vi "fft_test.vi"() -> ()   [LabVIEW 2012]
uses:
  <vilib>/express/express analysis/Spectral/Block/exnSpectralBlock spectral measurements peak poly.vi
  <vilib>/express/express analysis/Spectral/Block/exnSpectralBlock spectral measurements peak DDT.vi
  <vilib>/express/express analysis/Spectral/XNode/ExpressSpectralMeasurementsBlockNode.xnode
panel:
  out "data":dynamicdata(graph) caption="Daten"
  out "Signalverlaufsgraph":dynamicdata(graph)
  in  "stop (F)":bool caption="Stopp (F)"
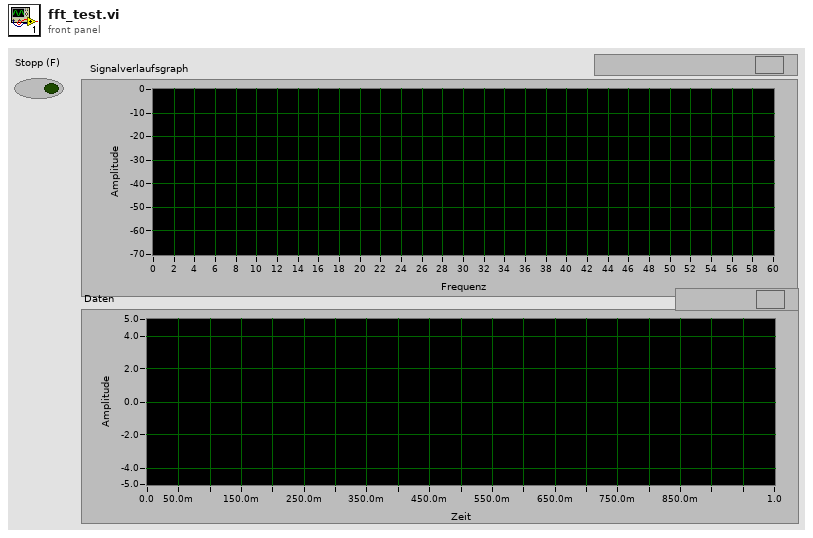
[diagram p1: front panel]
types:
  T1 = cluster{"averaging mode":u16, "weighting mode":u16, "number of averages":u32}
  T2 = cluster{"dB On (F)":bool, "unwrap phase (F)":bool, "convert to degree (F)":bool}
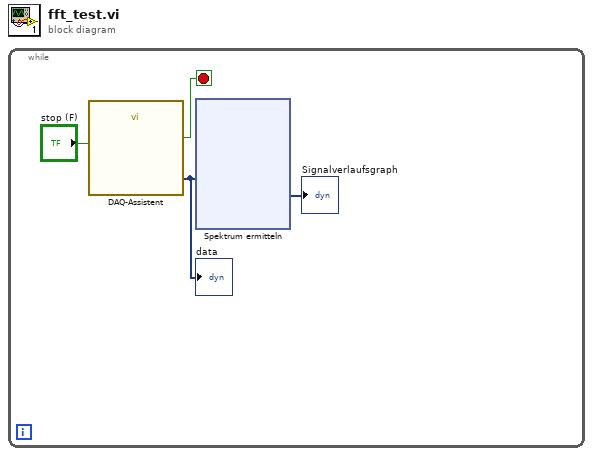
[diagram p0: block diagram]
diagram:
  n1 = while {
    stop <- w3 stop-if-true
    n2 = call "DAQ-Assistent"("stop (F)"="stop (F)") -> ("data"=w2:dynamicdata, "stopped"=w3:bool)  [unwired: 15 in, 2 out]
    "data" <- w2
    n3 = xnode "Spektrum ermitteln"("Signale"=w2) -> ("FFT - (Spitze)"=→"Signalverlaufsgraph":dynamicdata)  [unwired: 1 in, 2 out]
  }
